vi "Get Last Reading.vi"(8 "error in":errorcluster, 10 "Channel":string, 11 "BufferLastReads in":refnum<class "BufferLastReads.lvclass">) -> (0 "error out":errorcluster, 2 "Last Read":variant, 3 "BufferLastReads out":refnum<class "BufferLastReads.lvclass">)   [LabVIEW 2024, in "BufferLastReads.lvclass"]
uses:
  BufferLastReads.lvclass
  BufferLastReads.lvclass/BufferLastReads.ctl
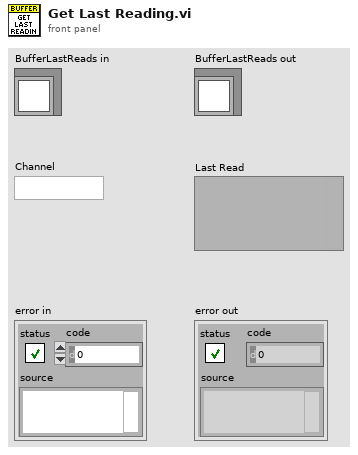
[diagram p1: front panel]
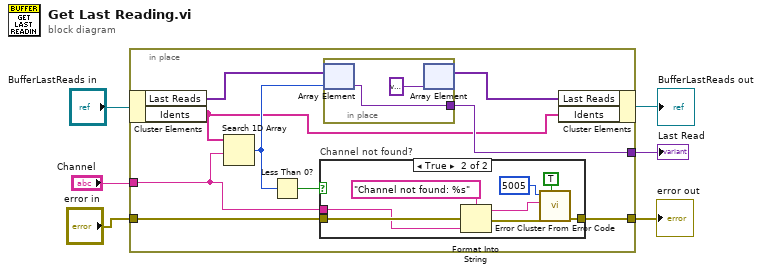
[diagram p0: block diagram]
diagram:
  n1 = in-place {
    in-place-border: [w8] -> w4
    in-place-border: [w15] -> w3
    in-place-border: "Channel" -> [w14]
    in-place-border: "error in" -> [w11]
    n2 = in-place-cluster #1("BufferLastReads in") -> ("Last Reads"=w10:variant[], "Idents"=w7:string[])
    n3 = Search 1D Array(1D array=w7, element=w14) -> (index of element=w12:i32)  [unwired: 1 in]
    n4 = Less Than 0?(x=w12) -> (x < 0?=w13:bool)
    n5 = case "Channel not found?" shown="True" w13 {
      tunnel: [w16 w23] -> w15
      tunnel: w11 -> [w16 w21]
      tunnel: w14 -> [_ w18]
      frame False {
      }
      frame True {
        n6 = Format Into String(format string="Channel not found: %s", error in=w21, w18) -> (resulting string=w17:string, error out=w20:errorcluster)  [unwired: 1 in]
        n7 = call <vilib>:"Error Cluster From Error Code.vi"("show call chain? (False)"=TRUE, "error in (no error)"=w20, "error message (\"\")"=w17, "error code (0)"=5005) -> ("error out"=w23:errorcluster)  [unwired: 5 in]
      }
    }
    n8 = in-place {
      in-place-border: [w25] -> w8
      n9 = in-place-array #2(w10, w12) -> (w25:variant)
      n10 = in-place-array #2(variant) -> (w9:variant[])  [unwired: 1 out]
    }
    n11 = in-place-cluster #1("Last Reads"=w9, "Idents"=w7) -> (→"BufferLastReads out":refnum<class "BufferLastReads.lvclass">)
  }
  "error out" <- w3
  "Last Read" <- w4
